vi "setOptionsString.vi"(8 "error in (no error)":errorcluster, 10 "OptionsString":string, 11 "tBSONRegEx in":refnum<class "tBSONRegEx.lvclass">) -> (0 "error out":errorcluster, 3 "tBSONRegEx out":refnum<class "tBSONRegEx.lvclass">)   [LabVIEW 2013, in "BSON.lvlib" / "tBSONRegEx.lvclass"]
uses:
  tBSONRegEx.lvclass
  options.ctl
  setOptions.vi
  <vilib>/regexp/Match Regular Expression.xnode
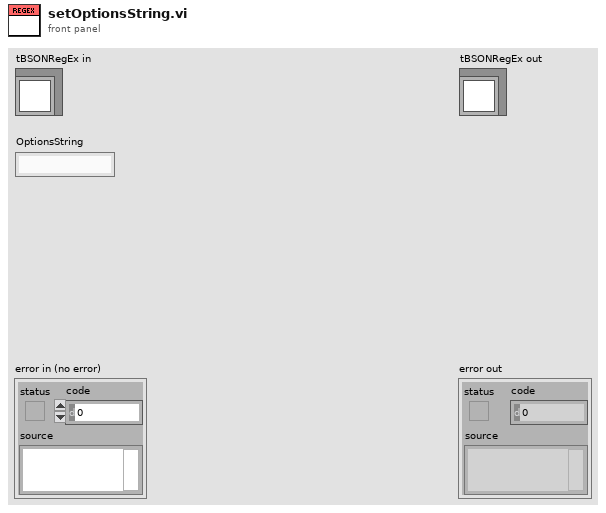
[diagram p1: front panel]
types:
  T1 = typedef "BSON.lvlib/tBSONRegEx.lvclass/options.ctl" = cluster{"Case Insensitive":bool, "Multiple Matching":bool, "Verbose Mode":bool, "Make \\w, \\W Local Dependent":bool, "Dotall mode":bool, "Make \\w, \\W Match Unicode":bool}
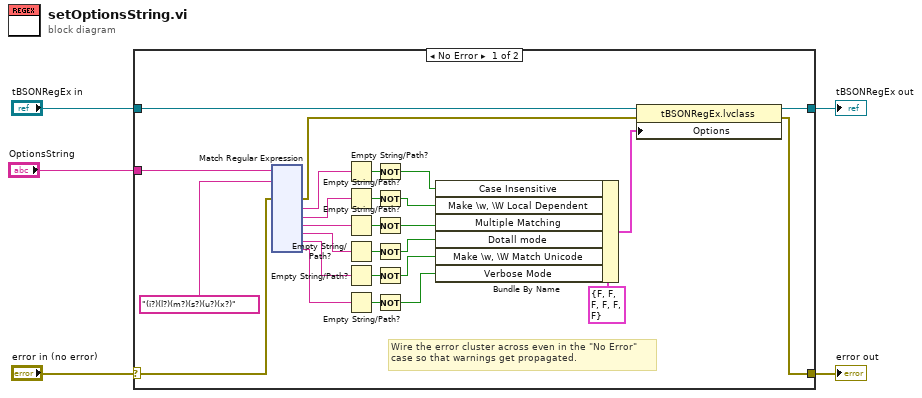
[diagram p0: block diagram]
diagram:
  n1 = case shown="No Error" "error in (no error)" {
    selector: "error in (no error)" -> [w9 w152]
    tunnel: [w10 w152] -> w4
    tunnel: [w11 w151] -> w2
    tunnel: "tBSONRegEx in" -> [w12 w151]
    tunnel: "OptionsString" -> [w6 _]
    frame No Error {
      # "Wire the error cluster across even in the \"No Error\"\ncase so that warnings get propagated."
      n2 = xnode "Match Regular Expression"("input string"=w6, "regular expression"="(i?)(l?)(m?)(s?)(u?)(x?)", "error in"=w9) -> ("error out"=w8:errorcluster, "submatch 1"=w22:string, "submatch 2"=w23:string, "submatch 3"=w24:string, "submatch 4"=w25:string, "submatch 5"=w26:string, "submatch 6"=w27:string)  [unwired: 3 in, 4 out]
      n3 = Empty String/Path?(string/path=w22) -> (empty?=w15:bool)
      n4 = Empty String/Path?(string/path=w23) -> (empty?=w17:bool)
      n5 = Empty String/Path?(string/path=w24) -> (empty?=w18:bool)
      n6 = Empty String/Path?(string/path=w25) -> (empty?=w19:bool)
      n7 = Empty String/Path?(string/path=w26) -> (empty?=w20:bool)
      n8 = Empty String/Path?(string/path=w27) -> (empty?=w21:bool)
      n9 = Not(x=w15) -> (.not. x?=w16:bool)
      n10 = Not(x=w17) -> (.not. x?=w28:bool)
      n11 = Not(x=w18) -> (.not. x?=w29:bool)
      n12 = Not(x=w19) -> (.not. x?=w30:bool)
      n13 = Not(x=w20) -> (.not. x?=w31:bool)
      n14 = Not(x=w21) -> (.not. x?=w32:bool)
      n15 = Bundle By Name(cluster=T1 {"Case Insensitive"=FALSE, "Multiple Matching"=FALSE, "Verbose Mode"=FALSE, "Make \\w, \\W Local Dependent"=FALSE, "Dotall mode"=FALSE, "Make \\w, \\W Match Unicode"=FALSE} ("Options"), "Case Insensitive"=w16, "Make \\w, \\W Local Dependent"=w28, "Multiple Matching"=w29, "Dotall mode"=w30, "Make \\w, \\W Match Unicode"=w31, "Verbose Mode"=w32) -> (w14:T1)
      n16 = property class="tBSONRegEx.lvclass"(reference=w12, error in=w8, "Options"=w14) -> (reference out=w11:refnum<class "tBSONRegEx.lvclass">, error out=w10:errorcluster)
    }
    frame Error {
    }
  }
  "error out" <- w4
  "tBSONRegEx out" <- w2
